vi "Pomiar diody.vi"() -> ()   [LabVIEW 2018]
panel:
  out "Napiecie na diodzie [V]":dbl
  out "Nr pomiaru":i32
  out "read buffer 4":string
  in  "Reset":bool
  out "XY Graph":cluster{"X":dbl[], "Y":dbl[]}[](graph)
  out "Boolean 2":bool
  out "Boolean":bool
  out "Prad [A]":dbl
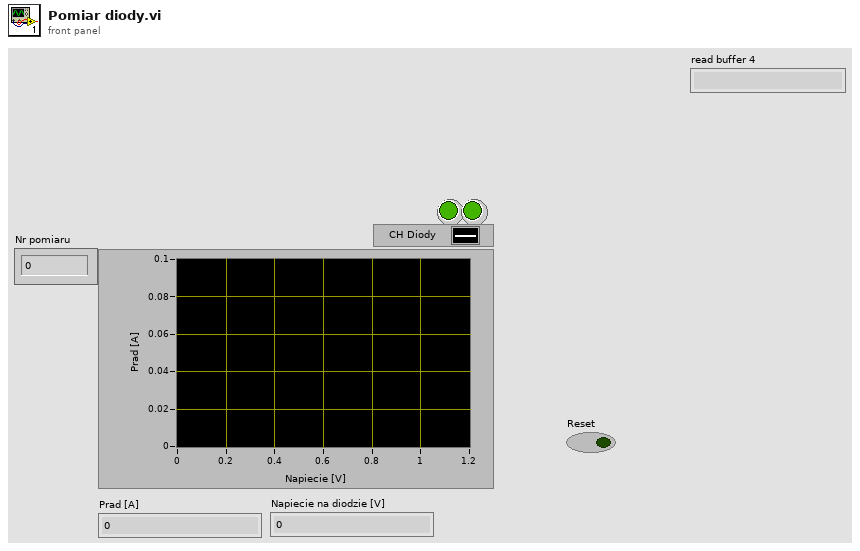
[diagram p1: front panel]
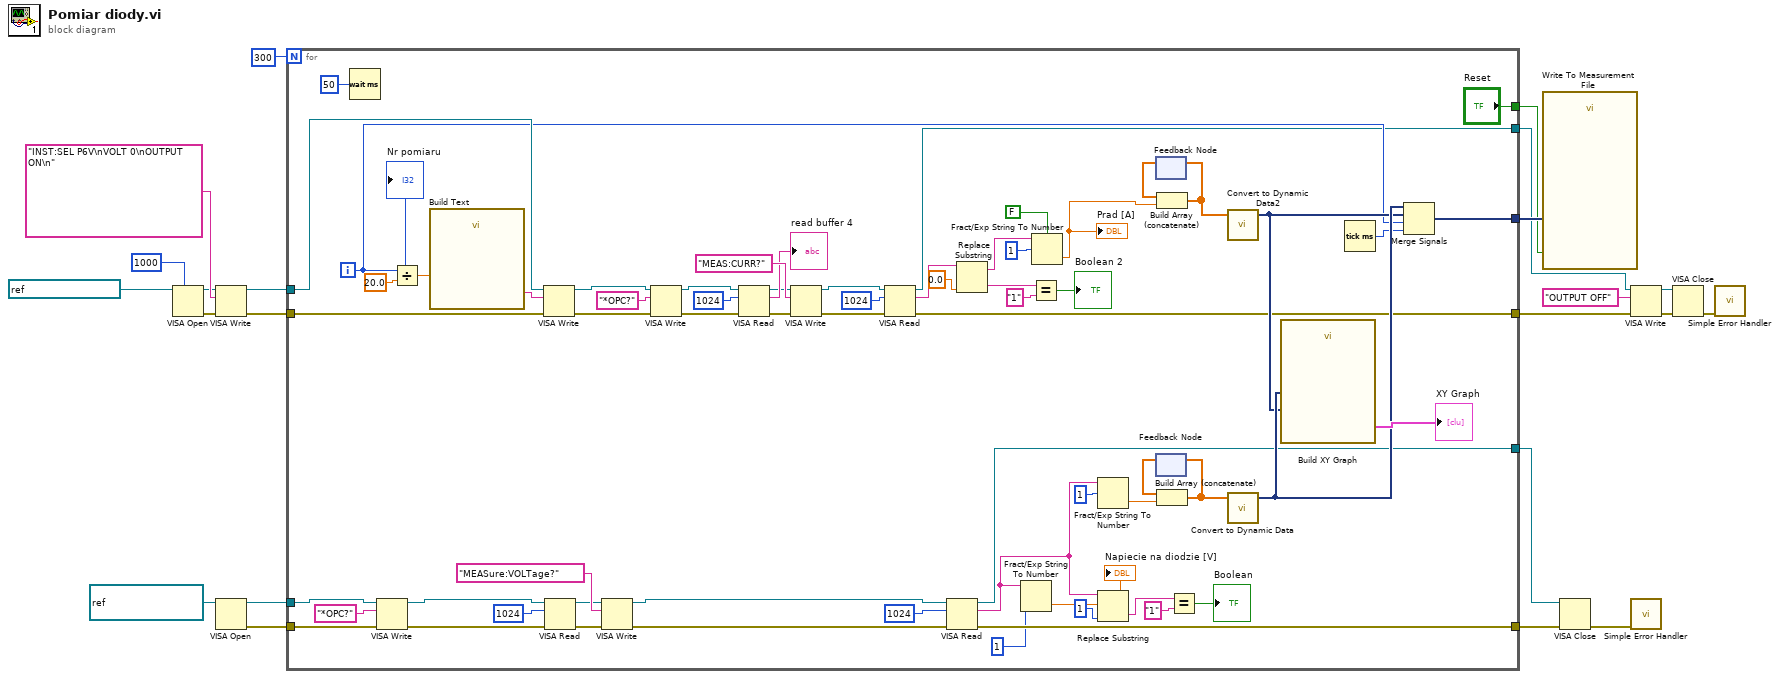
[diagram p0: block diagram]
diagram:
  n1 = VISA Open(timeout (0)=u32 1000 ("VISA Open timeout (0)"), VISA resource name=refnum<visa-resource-name> "GPIB0::9::INSTR") -> (VISA resource name=w15:refnum<visa-resource-name>, error out=w17:errorcluster)  [unwired: 3 in]
  n2 = VISA Write(VISA resource name=w15, write buffer="INST:SEL P6V\nVOLT 0\nOUTPUT ON\n", error in (no error)=w17) -> (VISA resource name out=w13:refnum<visa-resource-name>, error out=w14:errorcluster)  [unwired: 1 out]
  n3 = VISA Open(VISA resource name=refnum<visa-resource-name> "GPIB0::10::INSTR") -> (VISA resource name=w22:refnum<visa-resource-name>, error out=w21:errorcluster)  [unwired: 4 in]
  n4 = for {
    N: 300 -> [_]
    tunnel: w22 -> [w35]
    tunnel: w21 -> [w34]
    tunnel: w14 -> [w61]
    tunnel: w13 -> [w60]
    tunnel: [w52] -> w12
    tunnel: ["Reset"] -> w11
    tunnel: [w39] -> w9
    tunnel: [w38] -> w7
    tunnel: [w29] -> w4
    tunnel: [w28] -> w3
    i -> [w54]
    n5 = Wait (ms)(milliseconds to wait=u32 50) -> ()  [unwired: 1 out]
    n6 = VISA Write(VISA resource name=w35, write buffer="*OPC?", error in (no error)=w34) -> (VISA resource name out=w37:refnum<visa-resource-name>, error out=w36:errorcluster)  [unwired: 1 out]
    n7 = Divide(x=w54, y=20.0) -> (x/y=w72:dbl)
    n8 = call "Build Text"("d"=w72) -> ("Result"=w64:string)  [unwired: 13 in, 1 out]
    n9 = VISA Write(VISA resource name=w60, write buffer=w64, error in (no error)=w61) -> (VISA resource name out=w44:refnum<visa-resource-name>, error out=w46:errorcluster)  [unwired: 1 out]
    n10 = VISA Read(VISA resource name=w37, byte count=u32 1024, error in (no error)=w36) -> (VISA resource name out=w31:refnum<visa-resource-name>, error out=w30:errorcluster)  [unwired: 2 out]
    n11 = VISA Write(VISA resource name=w31, write buffer="MEASure:VOLTage?", error in (no error)=w30) -> (VISA resource name out=w33:refnum<visa-resource-name>, error out=w32:errorcluster)  [unwired: 1 out]
    n12 = VISA Write(VISA resource name=w44, write buffer="*OPC?", error in (no error)=w46) -> (VISA resource name out=w43:refnum<visa-resource-name>, error out=w42:errorcluster)  [unwired: 1 out]
    n13 = VISA Read(VISA resource name=w43, byte count=u32 1024, error in (no error)=w42) -> (VISA resource name out=w40:refnum<visa-resource-name>, read buffer=→"read buffer 4":string, error out=w41:errorcluster)  [unwired: 1 out]
    n14 = VISA Write(VISA resource name=w40, write buffer="MEAS:CURR?", error in (no error)=w41) -> (VISA resource name out=w27:refnum<visa-resource-name>, error out=w58:errorcluster)  [unwired: 1 out]
    n15 = VISA Read(VISA resource name=w27, byte count=u32 1024, error in (no error)=w58) -> (VISA resource name out=w38:refnum<visa-resource-name>, read buffer=w62:string, error out=w39:errorcluster)  [unwired: 1 out]
    n16 = VISA Read(VISA resource name=w33, byte count=u32 1024, error in (no error)=w32) -> (VISA resource name out=w28:refnum<visa-resource-name>, read buffer=w25:string, error out=w29:errorcluster)  [unwired: 1 out]
    n17 = Replace Substring(2:0.0, 5:w62) -> (0:w84:string, 1:w85:string)  [unwired: 2 in]
    n18 = Fract/Exp String To Number(string=w25, offset=1) -> (number=→"Napiecie na diodzie [V]":dbl)  [unwired: 2 in, 1 out]
    n19 = Equal?(x=w84, y="1") -> (x = y?=→"Boolean 2":bool)
    n20 = Fract/Exp String To Number(use system decimal point (T)=FALSE, string=w85, offset=1) -> (number=w66:dbl)  [unwired: 1 in, 1 out]
    "Prad [A]" <- w66
    n21 = Fract/Exp String To Number(string=w25, offset=1) -> (number=w68:dbl)  [unwired: 2 in, 1 out]
    n22 = Replace Substring(2:1 ("length (len. of substring)"), 5:w25) -> (0:w86:string)  [unwired: 2 in, 1 out]
    n23 = feedback #1() -> (w67:dbl[])  [unwired: 1 in]
    n24 = feedback #2() -> (w69:dbl[])  [unwired: 1 in]
    n25 = Build Array (concatenate)(w67, w66) -> (w65:dbl[])
    n26 = feedback-in #1(w65) -> ()
    n27 = Build Array (concatenate)(w69, w68) -> (w70:dbl[])
    n28 = feedback-in #2(w70) -> ()
    n29 = Equal?(x=w86, y="1") -> (x = y?=→"Boolean":bool)
    n30 = call "Convert to Dynamic Data2"("Array"=w65) -> ("Dynamic Data Type"=w55:dynamicdata)  [unwired: 3 in]
    n31 = call "Convert to Dynamic Data"("Array"=w70) -> ("Dynamic Data Type"=w56:dynamicdata)  [unwired: 3 in]
    n32 = call "Build XY Graph"("Y Input"=w55, "X Input"=w56) -> ("XY Graph"=→"XY Graph":cluster{"X":dbl[], "Y":dbl[]}[])  [unwired: 8 in, 1 out]
    n33 = Tick Count (ms)() -> (millisecond timer value=w53:u32)
    n34 = Merge Signals(w56, w55, w54, w53) -> (w52:dynamicdata)
    "Nr pomiaru" <- w54
  }
  n35 = call "Write To Measurement File"("Signals"=w12, "Reset"=w11) -> ()  [unwired: 15 in, 3 out]
  n36 = VISA Close(VISA resource name=w3, error in (no error)=w4) -> (error out=w2:errorcluster)
  n37 = VISA Write(VISA resource name=w7, write buffer="OUTPUT OFF", error in (no error)=w9) -> (VISA resource name out=w5:refnum<visa-resource-name>, error out=w6:errorcluster)  [unwired: 1 out]
  n38 = call <vilib>:"Simple Error Handler.vi"("error in (no error)"=w2) -> ()  [unwired: 4 in, 5 out]
  n39 = VISA Close(VISA resource name=w5, error in (no error)=w6) -> (error out=w10:errorcluster)
  n40 = call <vilib>:"Simple Error Handler.vi"("error in (no error)"=w10) -> ()  [unwired: 4 in, 5 out]
